vi "anglepidinit.vi"() -> ()   [LabVIEW 2013]
uses:
  <vilib>/addons/control/pid/pid.llb/PID (DBL).vi
  <vilib>/addons/control/pid/NI_PID_pid.lvlib
panel:
  in  "reinitialize? (F) 2":bool
  out "Done? 2":bool
  in  "Adjustment Variable 2":dbl=0.64
  in  "PID Gains for Angle":T1={"proportional gain (Kc)"=1.2, "integral time (Ti, min)"=0.011, "derivative time (Td, min)"=0.007} {"derivative time (Td, min)" format="%.3f"; "integral time (Ti, min)" format="%.3f"; "proportional gain (Kc)" format="%.3f"}
  in  "Angle Target":dbl
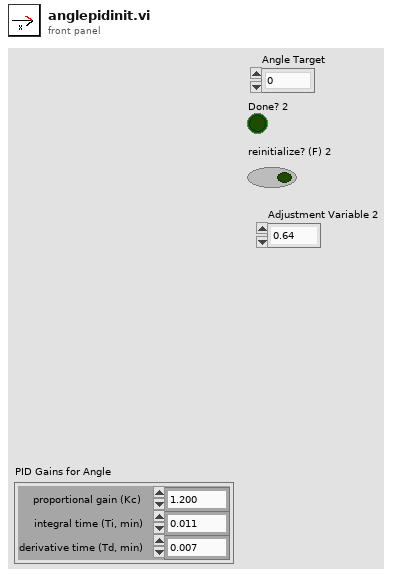
[diagram p1: front panel]
types:
  T1 = cluster{"proportional gain (Kc)":dbl, "integral time (Ti, min)":dbl, "derivative time (Td, min)":dbl}
  T2 = typedef "WPI_EncoderDevRef.ctl" = cluster{"DevStatus":errorcluster, "EncoderIndex":T3, "CounterIndex":T4, "DistancePerCount":dbl, "Decoding Type":T5}
  T3 = typedef "FPGA_EncoderIdx.ctl" = enum8{"Enc 0", "Enc 1", "Enc 2", "Enc 3", "Invalid"}
  T4 = typedef "FPGA_CounterCtrSystemIndex.ctl" = enum8{"Ctr 0", "Ctr 1", "Ctr 2", "Ctr 3", "Ctr 4", "Ctr 5", "Ctr 6", "Ctr 7", "Invalid"}
  T5 = typedef "WPI_EncoderType.ctl" = enum16{"1x", "2x", "4x"}
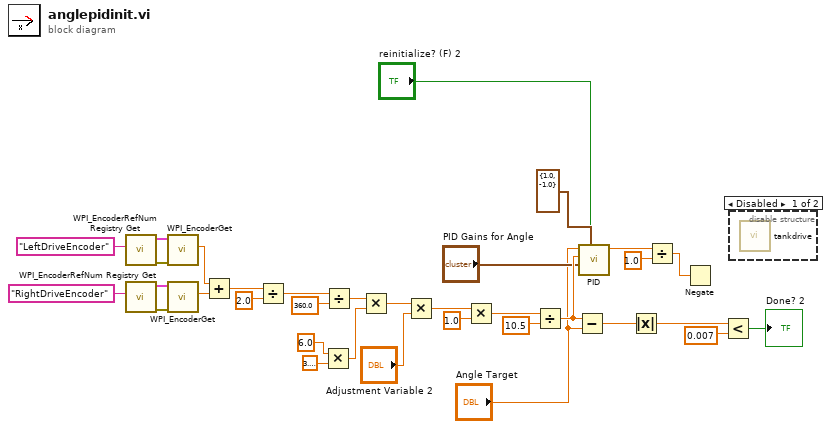
[diagram p0: block diagram]
diagram:
  n1 = call <vilib>:"WPI_EncoderRefNum Registry Get.vi"("refnum name"="LeftDriveEncoder") -> ("error out"=w34:errorcluster, "EncoderDevRef"=w33:T2)  [unwired: 9 in]
  n2 = call <vilib>:"WPI_EncoderRefNum Registry Get.vi"("refnum name"="RightDriveEncoder") -> ("error out"=w32:errorcluster, "EncoderDevRef"=w31:T2)  [unwired: 9 in]
  n3 = call <vilib>:"WPI_EncoderGet.vi"("error in (no error)"=w34, "EncoderDevRef"=w33) -> ("Distance"=w28:dbl)  [unwired: 4 in, 5 out]
  n4 = call <vilib>:"WPI_EncoderGet.vi"("error in (no error)"=w32, "EncoderDevRef"=w31) -> ("Distance"=w12:dbl)  [unwired: 4 in, 5 out]
  n5 = Add(x=w28, y=w12) -> (x+y=w27:dbl)
  n6 = Divide(x=w27, y=2.0) -> (x/y=w23:dbl)
  n7 = Multiply(x=6.0, y=3.141592653589793) -> (x*y=w21:dbl)
  n8 = Divide(x=w23, y=360.0) -> (x/y=w18:dbl)
  n9 = Multiply(x=w18, y=w21) -> (x*y=w9:dbl)
  n10 = Multiply(x=w9, y="Adjustment Variable 2") -> (x*y=w8:dbl)
  n11 = Multiply(x=w8, y=1.0) -> (x*y=w7:dbl)
  n12 = Divide(x=w7, y=10.5) -> (x/y=w14:dbl)
  n13 = Subtract(x=w14, y="Angle Target") -> (x-y=w15:dbl)
  n14 = call-poly <vilib>:"PID.vi"("reinitialize? (F)"="reinitialize? (F) 2", "output range"=cluster{"output high":dbl, "output low":dbl} {"output high"=1.0, "output low"=-1.0}, "PID gains"="PID Gains for Angle", "process variable"=w14, "setpoint"="Angle Target") -> ("output"=w19:dbl)  [unwired: 5 in, 1 out]
  n15 = Absolute Value(x=w15) -> (abs(x)=w16:dbl)
  n16 = Divide(x=w19, y=1.0) -> (x/y=w11:dbl)
  n17 = Negate(x=w11) -> ()  [unwired: 1 out]
  n18 = Less?(x=w16, y=0.007) -> (x < y?=→"Done? 2":bool)
  n19 = disable-structure shown="Disabled" {
    frame Disabled {
      n20 = call "tankdrive.vi"() -> ()  [unwired: 12 in]
    }
    frame Enabled {
    }
  }
